vi "MAX SWERVE.vi"() -> ()   [LabVIEW 2023]
uses:
  <vilib>/Rock Robotics/WPI/ThirdParty/REV Robotics/REVLib/Typedef/Spark MAX Sensor Type.ctl
  <vilib>/Rock Robotics/WPI/Joystick/WPI_JoystickDeviceEnum.ctl
  <vilib>/Rock Robotics/WPI/ThirdParty/REV Robotics/REVLib/Typedef/Spark MAX Control Type.ctl
panel:
  out "theta":dbl
  out "x*y":dbl
  out "Axes":dbl[](array[numeric])
  out "Sensor Velocity":dbl
  in  "PID Constants":T1={"P Gain"=0.0, "I Gain"=0.0, "D Gain"=0.0, "F Gain"=0.0, "I Zone"=0.0, "Min Output"=-1.0, "Max Output"=1.0}
  in  "stop":bool
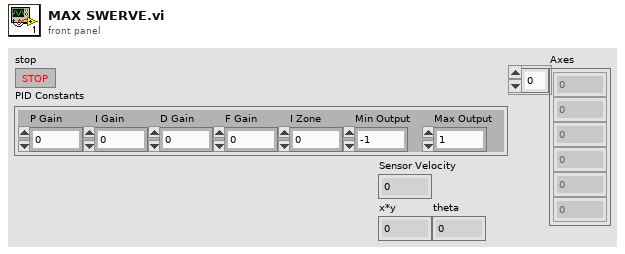
[diagram p1: front panel]
types:
  T1 = cluster{"P Gain":dbl, "I Gain":dbl, "D Gain":dbl, "F Gain":dbl, "I Zone":dbl, "Min Output":dbl, "Max Output":dbl}
  T2 = typedef "WPI_JoystickDeviceEnum.ctl" = enum16{"USB 0", "USB 1", "USB 2", "USB 3", "USB 4", "USB 5"}
  T3 = typedef "Spark MAX Sensor Type.ctl" = enum16{"No Sensor", "Hall Sensor", "Encoder", "-Not Available-", "Analog", "Alternate Encoder", "Duty Cycle"}
  T4 = typedef "WPI_MotorControlDeviceRef.ctl" = cluster{"DeviceStatus":errorcluster, "Type":T5, "PWM":cluster{"PWM Channel":T6, "DeadBand":T7}, "CAN":cluster{"Device Number":u8, "SetOutput VI Ref":variant, "GetOutput VI Ref":variant, "Enable VI Ref":variant, "Disable VI Ref":variant, "Data":variant}, "Invert":bool, "DIO PWM":cluster{"PWM \"Enable\" Channel":T6, "DIOChannel":T8, "PWM Rate":dbl}}
  T5 = typedef "WPI_MotorControlType.ctl" = enum16{"PWM", "CAN", "DIO PWM"}
  T6 = typedef "FPGA_DIOPWMChannel.ctl" = enum8{"PWM 0", "PWM 1", "PWM 2", "PWM 3", "PWM 4", "PWM 5", "PWM 6", "PWM 7", "PWM 8", "PWM 9", "PWM MXP 0", "PWM MXP 1", "PWM MXP 2", "PWM MXP 3", "PWM MXP 4", "PWM MXP 5", "PWM MXP 6", "PWM MXP 7", "PWM MXP 8", "PWM MXP 9", "Invalid"}
  T7 = typedef "WPI_PWMDeadband.ctl" = cluster{"Name":string, "maxPositivePwm":i32, "minPositivePwm":i32, "centerPwm":i32, "maxNegativePwm":i32, "minNegativePwm":i32, "angularRange":u16}
  T8 = typedef "FPGA_DIOChannel.ctl" = enum8{"DIO 0", "DIO 1", "DIO 2", "DIO 3", "DIO 4", "DIO 5", "DIO 6", "DIO 7", "DIO 8", "DIO 9", "DIO MXP 0", "DIO MXP 1", "DIO MXP 2", "DIO MXP 3", "DIO MXP 4", "DIO MXP 5", "DIO MXP 6", "DIO MXP 7", "DIO MXP 8", "DIO MXP 9", "DIO MXP 10", "DIO MXP 11", "DIO MXP 12", "DIO MXP 13", "DIO MXP 14", "DIO MXP 15", "SPI Port CS1", "SPI Port CS2", "SPI Port CS3", "SPI Port MISO", "SPI Port MOSI", "Invalid"}
  T9 = typedef "WPI_JoystickDevRef.ctl" = cluster{"Device":T2}
  T10 = typedef "Spark MAX Control Type.ctl" = enum16{"Percent VBus", "Voltage", "Velocity", "Position", "Smart Motion", "Current", "Smart Velocity"}
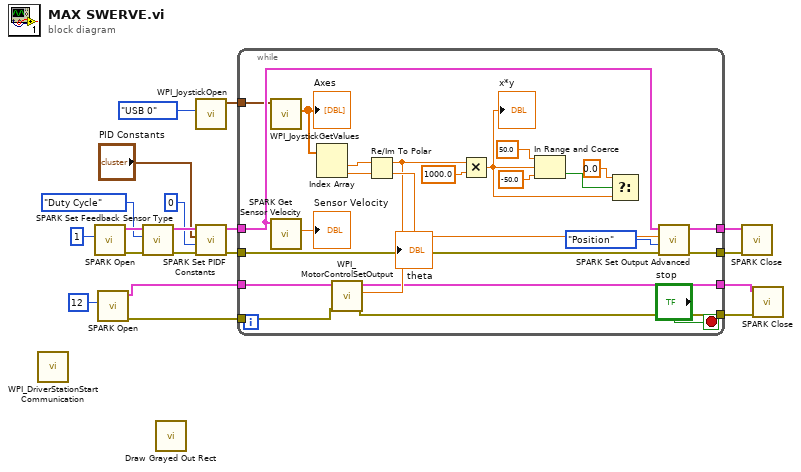
[diagram p0: block diagram]
diagram:
  n1 = call <vilib>:"WPI_DriverStationStart Communication.vi"() -> ()  [unwired: 12 in]
  n2 = call <vilib>:"SPARK Open.vi"("Device Number"=u8 1) -> ("error out"=w16:errorcluster, "MotorControlDeviceRef"=w18:T4)  [unwired: 9 in]
  n3 = call <vilib>:"SPARK Open.vi"("Device Number"=u8 12) -> ("error out"=w3:errorcluster, "MotorControlDeviceRef"=w4:T4)  [unwired: 9 in]
  n4 = call <vilib>:"SPARK Set Feedback Sensor Type.vi"("error in (no error)"=w16, "Sensor Type"=Spark_MAX_Sensor_Type."Duty Cycle", "MotorControlDevRef"=w18) -> ("error out"=w12:errorcluster, "MotorControlDeviceRef"=w15:T4)  [unwired: 7 in]
  n5 = call <vilib>:"Draw Grayed Out Rect.vi"() -> ()  [unwired: 5 in, 1 out]
  n6 = call <vilib>:"WPI_JoystickOpen.vi"("JoystickDevice"=WPI_JoystickDeviceEnum."USB 0") -> ("JoystickDevRef"=w6:T9)  [unwired: 10 in]
  n7 = call <vilib>:"SPARK Set PIDF Constants.vi"("error in"=w12, "PIDF Slot"=0, "PID Constants"="PID Constants", "MotorControlDeviceRef"=w15) -> ("error out"=w11:errorcluster, "MotorControlDeviceRef"=w10:T4)  [unwired: 6 in]
  n8 = while {
    tunnel: w11 -> [w41]
    tunnel: w10 -> [w37]
    tunnel: [w39] -> w9
    tunnel: [w38] -> w8
    tunnel: w6 -> [w35]
    tunnel: w4 -> [w24]
    tunnel: w3 -> [w23]
    tunnel: [w21] -> w2
    tunnel: [w20] -> w1
    stop <- "stop" stop-if-true
    n9 = call <vilib>:"WPI_JoystickGetValues.vi"("JoystickDevRef"=w35) -> ("Axes"=w34:dbl[])  [unwired: 6 in, 4 out]
    "Axes" <- w34
    n10 = call <vilib>:"SPARK Get Sensor Velocity.vi"("MotorControlDevRef in"=w37) -> ("Sensor Velocity"=→"Sensor Velocity":dbl)  [unwired: 7 in, 3 out]
    n11 = Index Array(array=w34) -> (element #1=w32:dbl, element #2=w33:dbl)  [unwired: 2 in]
    n12 = Re/Im To Polar(2:w33, 3:w32) -> (0:w25:dbl, 1:w22:dbl)
    "theta" <- w25
    n13 = call <vilib>:"WPI_MotorControlSetOutput.vi"("error in (no error)"=w23, "Output"=w22, "MotorControlDevRef"=w24) -> ("error out"=w21:errorcluster, "MotorControlDevRef"=w20:T4)  [unwired: 6 in, 1 out]
    n14 = Multiply(x=w22, y=1000.0) -> (x*y=w26:dbl)
    "x*y" <- w26
    n15 = In Range and Coerce(upper limit=50.0, x=w26, lower limit=-50.0) -> (In Range?=w28:bool)  [unwired: 1 out]
    n16 = Select(t=0.0, s=w28, f=w26) -> ()  [unwired: 1 out]
    n17 = call <vilib>:"SPARK Set Output Advanced.vi"("error in (no error)"=w41, "Control Mode"=Spark_MAX_Control_Type."Position", "Setpoint"=w25, "MotorControlDevRef"=w37) -> ("error out"=w39:errorcluster, "MotorControlDevRef"=w38:T4)  [unwired: 6 in]
  }
  n18 = call <vilib>:"SPARK Close.vi"("error in"=w9, "MotorControlDeviceRef"=w8) -> ()  [unwired: 9 in, 1 out]
  n19 = call <vilib>:"SPARK Close.vi"("error in"=w2, "MotorControlDeviceRef"=w1) -> ()  [unwired: 9 in, 1 out]
